vi "PrepChannelPlot.vi"(0 "Data In":dbl[][](array[numeric]), 1 "Plot Properties":T1 {"Zoom Factor" min=0.0 max=1.0}, 2 "Effective Sampling Rate":dbl, 3 "Error In":errorcluster, 4 "Init":bool=TRUE) -> (5 "Data Out":dbl[][](array[numeric]), 6 "Error Out":errorcluster)   [LabVIEW 2012]
uses:
  controls/PlotProperties.ctl
  <vilib>/Analysis/baseanly.llb/Mean (DBL).vi
  <vilib>/Analysis/NI_AALBase.lvlib
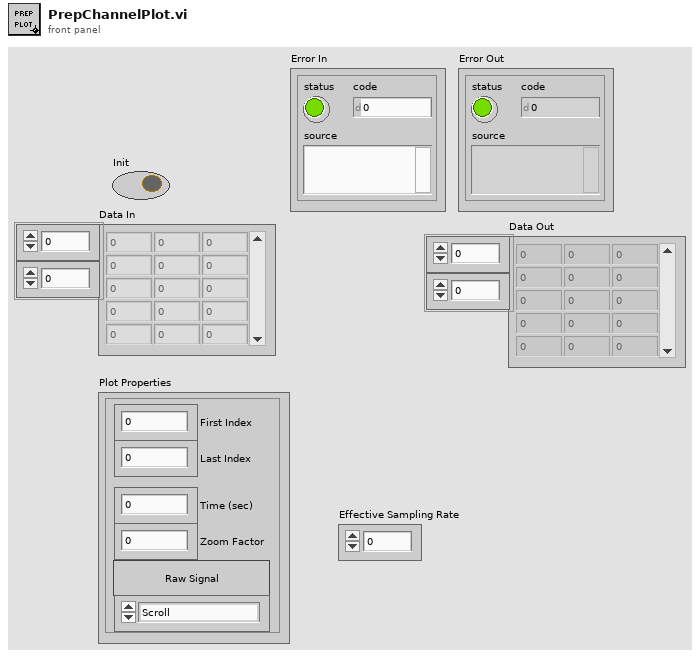
[diagram p1: front panel]
types:
  T1 = typedef "PlotProperties.ctl" = cluster{"First Index":i32, "Last Index":i32, "Time (sec)":dbl, "Zoom Factor":dbl, "SubtractMean?":bool, "DisplayOption":enum16{"Scroll", "Monitor"}}
  T2 = cluster{"First Index":bool, "Last Index":bool, "Time (sec)":bool, "Zoom Factor":bool, "SubtractMean?":bool, "DisplayOption":bool}
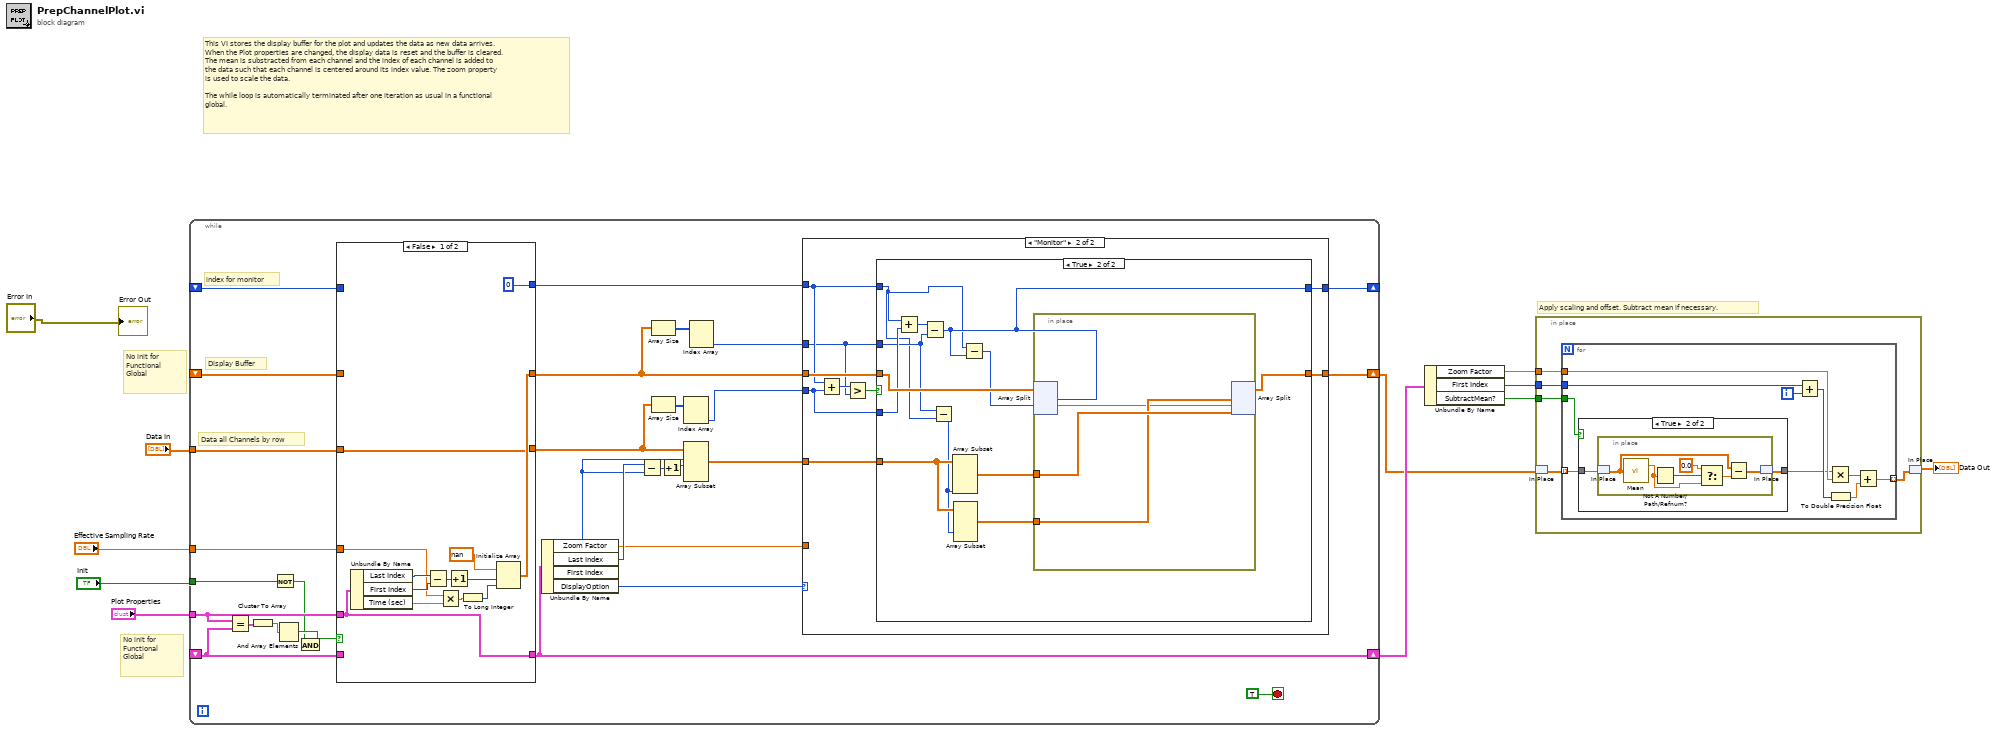
[diagram p0: block diagram]
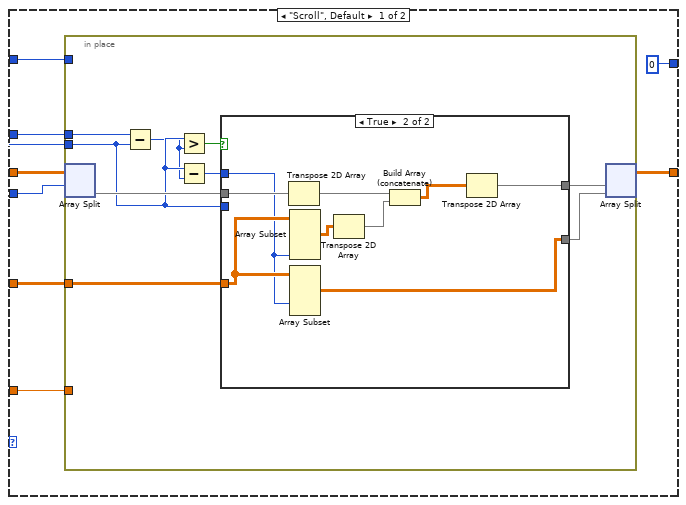
[diagram p3: hidden frame]
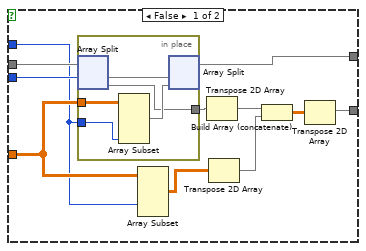
[diagram p4: hidden frame]
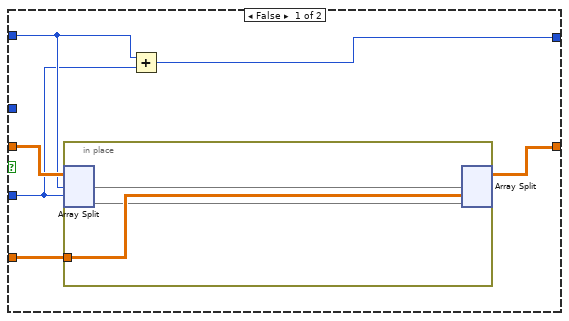
[diagram p5: hidden frame]
diagram:
  # "This VI stores the display buffer for the plot and updates the data as new data arrives.\nWhen the Plot properties are changed, the display data is reset and the buffer is cleared.\nThe mean is substracted from each channel and the index of each channel is added to \nthe data such that each channel is centered around its index value. The zoom property \nis used to scale the data.\n\nThe while loop is automatically terminated after one iteration as usual in a functional \nglobal."
  # "Apply scaling and offset. Subtract mean if necessary."
  # "No init for Functional Global"
  # "No init for Functional Global"
  n1 = while {
    tunnel: "Data In" -> [w33]
    tunnel: "Plot Properties" -> [w35]
    shift-right: [w16] -> w1
    shift-left: _ -> [w32]
    shift-right: [w17] -> w6
    shift-left: _ -> [w34]
    tunnel: "Effective Sampling Rate" -> [w21]
    tunnel: "Init" -> [w19]
    shift-right: [w12] -> _
    shift-left: _ -> [w15]
    stop <- TRUE stop-if-true
    # "index for monitor"
    # "Display Buffer"
    # "Data all Channels by row"
    n2 = Equal?(x=w35, y=w34) -> (x = y?=w37:T2)
    n3 = Cluster To Array(cluster=w37) -> (array=w38:bool[])
    n4 = Not(x=w19) -> (.not. x?=w18:bool)
    n5 = And Array Elements(Boolean array=w38) -> (logical AND=w36:bool)
    n6 = And(x=w36, y=w18) -> (x .and. y?=w20:bool)
    n7 = case shown="False" w20 {
      tunnel: w35 -> [w129 _]
      tunnel: w34 -> [_ w133]
      tunnel: [w129 w133] -> w17
      tunnel: w33 -> [w122 w131]
      tunnel: w32 -> [_ w132]
      tunnel: [w124 w132] -> w25
      tunnel: [w122 w131] -> w29
      tunnel: w21 -> [w120 _]
      tunnel: w15 -> [_ w130]
      tunnel: [0 w130] -> w14
      frame False {
        n8 = Unbundle By Name(w129) -> ("Last Index"=w128:i32, "First Index"=w127:i32, "Time (sec)"=w121:dbl)
        n9 = Subtract(x=w128, y=w127) -> (x-y=w126:i32)
        n10 = Multiply(x=w120, y=w121) -> (x*y=w119:dbl)
        n11 = Increment(x=w126) -> (x+1=w125:i32)
        n12 = To Long Integer(number=w119) -> (32bit integer=w118:i32)
        n13 = Initialize Array(nan, w125, w118) -> (w124:dbl[][])
      }
      frame True {
      }
    }
    n14 = Unbundle By Name(w17) -> ("Zoom Factor"=w26:dbl, "Last Index"=w31:i32, "First Index"=w27:i32, "DisplayOption"=w13:enum16{"Scroll", "Monitor"})
    n15 = Subtract(x=w31, y=w27) -> (x-y=w41:i32)
    n16 = Array Size(array=w25) -> (size(s)=w24:i32[])
    n17 = Array Size(array=w29) -> (size(s)=w30:i32[])
    n18 = Increment(x=w41) -> (x+1=w40:i32)
    n19 = Index Array(array=w30) -> (element #2=w28:i32)  [unwired: 2 in, 1 out]
    n20 = Array Subset(array=w29, index (row)=w27, length (row)=w40) -> (w22:dbl[][])  [unwired: 2 in]
    n21 = Index Array(array=w24) -> (element #2=w23:i32)  [unwired: 2 in, 1 out]
    n22 = case shown="\"Monitor\"" w13 {
      tunnel: w28 -> [w49 w87]
      tunnel: w26 -> [w48 _]
      tunnel: w25 -> [w47 w89]
      tunnel: w23 -> [w46 w84]
      tunnel: w22 -> [w45 w90]
      tunnel: [w44 w86] -> w16
      tunnel: w14 -> [w43 w88]
      tunnel: [0 w85] -> w12
      frame "Scroll", Default {
        n23 = in-place {
          in-place-border: w45 -> [w53]
          in-place-border: w49 -> [w55]
          in-place-border: w48 -> [_]
          in-place-border: w46 -> [w58]
          in-place-border: w43 -> [_]
          n24 = in-place-split #1(w47, w49) -> (w56:dbl[][])  [unwired: 1 out]
          n25 = Subtract(x=w58, y=w55) -> (x-y=w51:i32)
          n26 = Greater?(x=w55, y=w51) -> (0:w52:bool)
          n27 = Subtract(x=w55, y=w51) -> (x-y=w50:i32)
          n28 = case shown="True" w52 {
            tunnel: w53 -> [w66 w78]
            tunnel: [w67 w75] -> w57
            tunnel: [w59 w77] -> w54
            tunnel: w56 -> [w69 w83]
            tunnel: w50 -> [w65 w76]
            tunnel: w55 -> [w68 _]
            frame False {
              n29 = in-place {
                in-place-border: w66 -> [w74]
                in-place-border: w65 -> [w73]
                in-place-border: [w70] -> w62
                n30 = in-place-split #2(w69, w68) -> (w71:dbl[][], w70:dbl[][])
                n31 = Array Subset(array=w74, length (col)=w73) -> (w72:dbl[][])  [unwired: 3 in]
                n32 = in-place-split #2(w71, w72) -> (w67:dbl[][])  [unwired: 1 out]
              }
              n33 = Array Subset(array=w66, index (col)=w65) -> (w64:dbl[][])  [unwired: 3 in]
              n34 = Transpose 2D Array(2D array=w62) -> (transposed array=w61:dbl[][])
              n35 = Transpose 2D Array(2D array=w64) -> (transposed array=w63:dbl[][])
              n36 = Build Array (concatenate)(w61, w63) -> (w60:dbl[][])
              n37 = Transpose 2D Array(2D array=w60) -> (transposed array=w59:dbl[][])
            }
            frame True {
              n38 = Transpose 2D Array(2D array=w83) -> (transposed array=w81:dbl[][])
              n39 = Array Subset(array=w78, length (col)=w76) -> (w80:dbl[][])  [unwired: 3 in]
              n40 = Array Subset(array=w78, index (col)=w76) -> (w77:dbl[][])  [unwired: 3 in]
              n41 = Transpose 2D Array(2D array=w80) -> (transposed array=w79:dbl[][])
              n42 = Build Array (concatenate)(w81, w79) -> (w82:dbl[][])
              n43 = Transpose 2D Array(2D array=w82) -> (transposed array=w75:dbl[][])
            }
          }
          n44 = in-place-split #1(w57, w54) -> (w44:dbl[][])  [unwired: 1 out]
        }
      }
      frame "Monitor" {
        n45 = Add(x=w88, y=w87) -> (x+y=w92:i32)
        n46 = Greater?(x=w92, y=w84) -> (0:w91:bool)
        n47 = case shown="True" w91 {
          tunnel: w90 -> [w97 w108]
          tunnel: w89 -> [w98 w113]
          tunnel: w88 -> [w95 w103]
          tunnel: w87 -> [w94 w105]
          tunnel: [w96 w107] -> w86
          tunnel: [w93 w106] -> w85
          tunnel: w84 -> [_ w104]
          frame False {
            n48 = in-place {
              in-place-border: w97 -> [w100]
              n49 = in-place-split #3(w98, w95, w94) -> (w101:dbl[][], w99:dbl[][])  [unwired: 1 out]
              n50 = in-place-split #3(w101, w100, w99) -> (w96:dbl[][])  [unwired: 2 out]
            }
            n51 = Add(x=w95, y=w94) -> (x+y=w93:i32)
          }
          frame True {
            n52 = Add(x=w103, y=w105) -> (x+y=w112:i32)
            n53 = Subtract(x=w112, y=w104) -> (x-y=w106:i32)
            n54 = Subtract(x=w104, y=w103) -> (x-y=w102:i32)
            n55 = Array Subset(array=w108, length (col)=w102) -> (w110:dbl[][])  [unwired: 3 in]
            n56 = Array Subset(array=w108, index (col)=w102) -> (w109:dbl[][])  [unwired: 3 in]
            n57 = Subtract(x=w103, y=w106) -> (x-y=w111:i32)
            n58 = in-place {
              in-place-border: w110 -> [w116]
              in-place-border: w109 -> [w115]
              n59 = in-place-split #4(w113, w106, w111) -> (w114:dbl[][])  [unwired: 2 out]
              n60 = in-place-split #4(w115, w114, w116) -> (w107:dbl[][])  [unwired: 2 out]
            }
          }
        }
      }
    }
  }
  n61 = Unbundle By Name(w6) -> ("Zoom Factor"=w4:dbl, "First Index"=w5:i32, "SubtractMean?"=w3:bool)
  n62 = in-place {
    in-place-border: w5 -> [w138]
    in-place-border: w4 -> [w137]
    in-place-border: w3 -> [w136]
    n63 = in-place-match #5(w1) -> (w134:dbl[][])
    n64 = for {
      tunnel: w134 -> [w140] mode=indexing
      tunnel: w138 -> [w147]
      tunnel: [w144] -> w135 mode=indexing
      tunnel: w137 -> [w143]
      tunnel: w136 -> [w141]
      i -> [w148]
      n65 = case shown="True" w141 {
        tunnel: w140 -> [w149 w151]
        tunnel: [w149 w150] -> w139
        frame False {
        }
        frame True {
          n66 = in-place {
            n67 = in-place-match #6(w151) -> (w153:dbl[])
            n68 = call-poly <vilib>:"Mean.vi"("X"=w153) -> ("mean"=w156:dbl)  [unwired: 1 out]
            n69 = Not A Number/Path/Refnum?(number/path/refnum=w156) -> (NaN/Path/Refnum?=w157:bool)
            n70 = Select(t=0.0, s=w157, f=w156) -> (s? t:f=w154:dbl)
            n71 = Subtract(x=w153, y=w154) -> (x-y=w152:dbl[])
            n72 = in-place-match #6(w152) -> (w150:dbl[])
          }
        }
      }
      n73 = Add(x=w147, y=w148) -> (x+y=w146:i32)
      n74 = Multiply(x=w139, y=w143) -> (x*y=w142:dbl[])
      n75 = To Double Precision Float(number=w146) -> (double precision float=w145:dbl)
      n76 = Add(x=w142, y=w145) -> (x+y=w144:dbl[])
    }
    n77 = in-place-match #5(w135) -> (→"Data Out":dbl[][])
  }
  "Error Out" <- "Error In"
